vi "PCAN_DecompMessage.vi"(11 "CAN_Message out":T1) -> (0 "Detector4 Shutter Open?":bool, 1 "Detector3 Shutter Open?":bool, 2 "Detector2 Shutter Open?":bool, 3 "Detector1 Shutter Open?":bool, 4 "Laser 1-4":u8[](array[numeric]), 5 "Excitation Shutter Open?":bool, 6 "Laser 5-8":u8[](array[numeric]), 7 "Intensity (a.u.)":dbl)   [LabVIEW 2010]
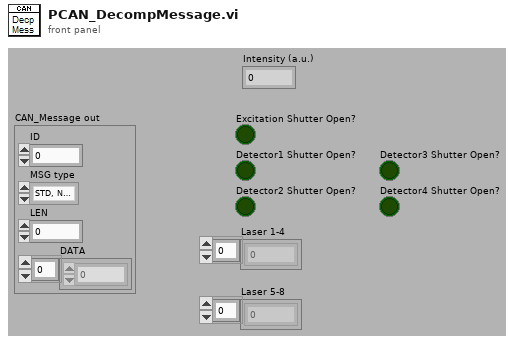
[diagram p1: front panel]
types:
  T1 = cluster{"ID":u32, "MSG type":enum8{"STD, NO RTR", "STD,RTR", "XTD, NO RTR", "XTD, RTR"}, "LEN":u8, "DATA":u8[]}
  T2 = enum8{"STD, NO RTR", "STD,RTR", "XTD, NO RTR", "XTD, RTR"}
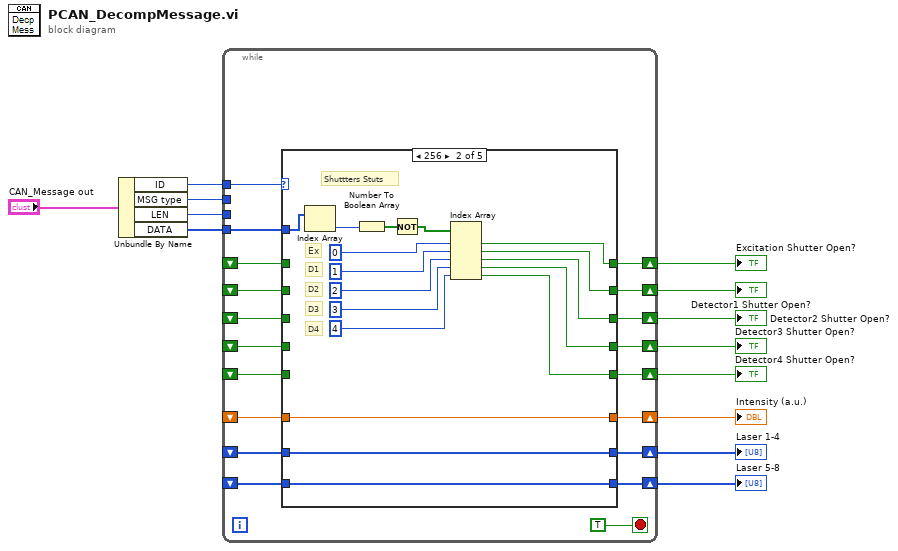
[diagram p0: block diagram]
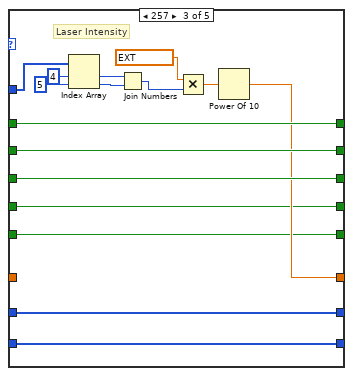
[diagram p3: hidden frame]
diagram:
  n1 = Unbundle By Name("CAN_Message out") -> ("ID"=w12:u32, "MSG type"=w11:T2, "LEN"=w10:u8, "DATA"=w9:u8[])
  n2 = while {
    tunnel: w12 -> [w31]
    tunnel: w11 -> [_]
    tunnel: w10 -> [_]
    tunnel: w9 -> [w30]
    shift-right: [w29] -> w7
    shift-left: _ -> [w24]
    shift-right: [w28] -> w6
    shift-left: _ -> [w25]
    shift-right: [w27] -> w8
    shift-left: _ -> [w26]
    shift-right: [w23] -> w5
    shift-left: _ -> [w22]
    shift-right: [w21] -> w4
    shift-left: _ -> [w20]
    shift-right: [w19] -> w3
    shift-left: _ -> [w18]
    shift-right: [w16] -> w1
    shift-left: _ -> [w15]
    shift-right: [w17] -> w2
    shift-left: _ -> [w14]
    stop <- TRUE stop-if-true
    n3 = case shown="256" w31 {
      tunnel: w30 -> [_ w57 w70 w77 w84]
      tunnel: [w38 w45 w71 w79 w87] -> w29
      tunnel: [w39 w44 w72 w80 w88] -> w28
      tunnel: [w40 w43 w73 w81 w89] -> w27
      tunnel: w26 -> [w40 _ w73 w81 w89]
      tunnel: w25 -> [w39 _ w72 w80 w88]
      tunnel: w24 -> [w38 _ w71 w79 w87]
      tunnel: [w37 w56 w63 w78 w86] -> w23
      tunnel: w22 -> [w37 w56 _ w78 w86]
      tunnel: [w36 w55 w61 w77 w85] -> w21
      tunnel: w20 -> [w36 w55 w61 _ w85]
      tunnel: [w35 w54 w60 w76 w84] -> w19
      tunnel: w18 -> [w35 w54 w60 w76 _]
      tunnel: [w33 w42 w58 w75 w82] -> w17
      tunnel: [w34 w41 w59 w74 w83] -> w16
      tunnel: w15 -> [w34 _ w59 w74 w83]
      tunnel: w14 -> [w33 _ w58 w75 w82]
      frame 0, Default {
      }
      frame 256 {
        # "D4"
        # "D3"
        # "Shuttters Stuts"
        # "D2"
        # "D1"
        # "Ex"
        n4 = Index Array(array=w57) -> (element=w53:u8)  [unwired: 1 in]
        n5 = Number To Boolean Array(number=w53) -> (Boolean array=w52:bool[])
        n6 = Not(x=w52) -> (.not. x?=w51:bool[])
        n7 = Index Array(array=w51, index #1=0 ("y"), index #2=1 ("y"), index #3=2 ("y"), index #4=3 ("y"), index #5=4 ("y")) -> (element #1=w43:bool, element #2=w44:bool, element #3=w45:bool, element #4=w41:bool, element #5=w42:bool)
      }
      frame 257 {
        # "Laser Intensity"
        n8 = Index Array(array=w70, index #1=4 ("index"), index #2=5 ("index")) -> (element #1=w67:u8, element #2=w66:u8)
        n9 = Join Numbers(hi=w67, lo=w66) -> ((hi.lo)=w62:u16)
        n10 = Multiply(x=ext 0.0097752, y=w62) -> (x*y=w64:ext)
        n11 = Power Of 10(x=w64) -> (10^x=w63:ext)
      }
      frame 1792 {
        # "Laser Controler 1"
      }
      frame 1793 {
        # "Laser Controler 2"
      }
    }
  }
  "Excitation Shutter Open?" <- w8
  "Detector2 Shutter Open?" <- w7
  "Detector1 Shutter Open?" <- w6
  "Intensity (a.u.)" <- w5
  "Laser 1-4" <- w4
  "Laser 5-8" <- w3
  "Detector4 Shutter Open?" <- w2
  "Detector3 Shutter Open?" <- w1
